vi "Lift Control.vi"(0 "Joystick Input":dbl, 1 "Lift Control":bool) -> ()   [LabVIEW 2014]
panel:
  out "error out motor lift":errorcluster
  out "Motor Output Lift":dbl
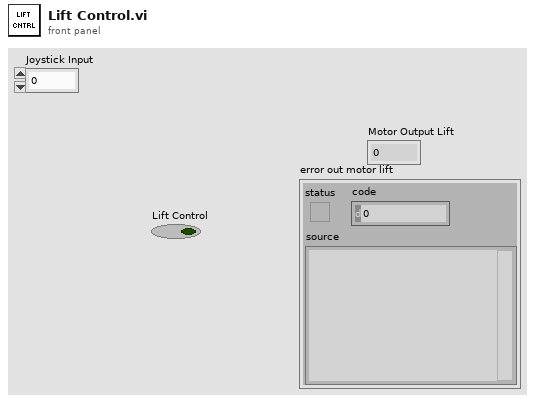
[diagram p1: front panel]
types:
  T1 = typedef "WPI_PotentiometerDevRef.ctl" = cluster{"DevStatus":errorcluster, "Controller":T2, "Analog Channel":T3, "Invert Output":bool}
  T2 = typedef "FPGA_TypedefAnalogModule.ctl" = enum16{"Controller 1"}
  T3 = typedef "FPGA_AIChannel.ctl" = enum8{"AI 0", "AI 1", "AI 2", "AI 3", "AI MXP 0", "AI MXP 1", "AI MXP 2", "AI MXP 3", "Invalid"}
  T4 = typedef "WPI_MotorControlDeviceRef.ctl" = cluster{"DeviceStatus":errorcluster, "Type":T5, "PWM":cluster{"Controller":T6, "PWM Channel":T7, "DeadBand":T8}, "CAN":cluster{"Device Number":u8, "Control Mode":T9, "Semaphore":T10, "Max Vout":dbl, "TalonSRX Control Mode":T11}, "Invert":bool, "TransformRef":T12, "InvTransformRef":T12}
  T5 = typedef "WPI_MotorControlType.ctl" = enum16{"PWM", "CAN", "CANTalonSRX"}
  T6 = typedef "FPGA_TypedefDigitalModule.ctl" = enum16{"Controller 1"}
  T7 = typedef "FPGA_DIOPWMChannel.ctl" = enum8{"PWM 0", "PWM 1", "PWM 2", "PWM 3", "PWM 4", "PWM 5", "PWM 6", "PWM 7", "PWM 8", "PWM 9", "PWM MXP 0", "PWM MXP 1", "PWM MXP 2", "PWM MXP 3", "PWM MXP 4", "PWM MXP 5", "PWM MXP 6", "PWM MXP 7", "PWM MXP 8", "PWM MXP 9", "Invalid"}
  T8 = typedef "WPI_PWMDeadband.ctl" = cluster{"Name":string, "maxPositivePwm":i32, "minPositivePwm":i32, "centerPwm":i32, "maxNegativePwm":i32, "minNegativePwm":i32, "angularRange":u16}
  T9 = typedef "WPI_CANJaguar_ControlMode.ctl" = enum8{"Percent VBus", "Current", "Speed", "Position", "Voltage"}
  T10 = typedef "Semaphore RefNum" = refnum<k1>
  T11 = typedef "WPI_CANTalonSRX_APIControlMode.ctl" = enum8{"Percent VBus", "Speed", "Position", "Slave", "Unchanged / Invalid"}
  T12 = typedef "WPI_PWMTransform_ConPane.ctl" = refnum<vi>
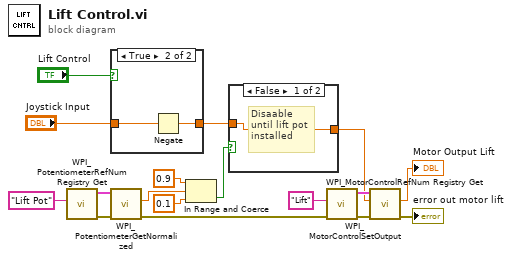
[diagram p0: block diagram]
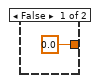
[diagram p3: hidden frame]
diagram:
  n1 = call <vilib>:"WPI_PotentiometerRefNum Registry Get.vi"("refnum name"="Lift Pot") -> ("error out"=w10:errorcluster, "PotDevRef"=w11:T1)  [unwired: 9 in]
  n2 = case shown="True" "Lift Control" {
    tunnel: "Joystick Input" -> [_ w20]
    tunnel: [0.0 ("Output") w19] -> w4
    frame False {
    }
    frame True {
      n3 = Negate(x=w20) -> (-x=w19:dbl)
    }
  }
  n4 = call <vilib>:"WPI_PotentiometerGetNormalized.vi"("error in"=w10, "PotDevRef"=w11) -> ("error out"=w2:errorcluster, "Normalized Value"=w7:dbl)  [unwired: 7 in, 1 out]
  n5 = In Range and Coerce(upper limit=0.9, x=w7, lower limit=0.1) -> (In Range?=w6:bool)  [unwired: 1 out]
  n6 = case shown="False" w6 {
    tunnel: [w21 w22] -> w5
    tunnel: w4 -> [w21 w22]
    frame False {
      # "Disaable\nuntil lift pot\ninstalled"
    }
    frame True {
    }
  }
  n7 = call <vilib>:"WPI_MotorControlRefNum Registry Get.vi"("error in (no error)"=w2, "refnum name"="Lift") -> ("error out"=w13:errorcluster, "MotorControlDevRef"=w14:T4)  [unwired: 8 in]
  n8 = call <vilib>:"WPI_MotorControlSetOutput.vi"("error in (no error)"=w13, "Output"=w5, "MotorControlDevRef"=w14) -> ("error out"=→"error out motor lift":errorcluster, "Motor Output"=→"Motor Output Lift":dbl)  [unwired: 6 in, 1 out]
